vi "Send Delayed Set DER Control.vi"(5 "Message Type":refnum<class "Set DER Control Msg.lvclass">, 7 "Message Priority (Normal)":T3=enum."Normal", 8 "error in (no error)":errorcluster, 9 "Milliseconds To Wait":i32=1000, 10 "DER_Control":T1, 11 "Message Enqueuer":refnum<class "Message Enqueuer.lvclass">) -> (0 "error out":errorcluster, 3 "Message Enqueuer out":refnum<class "Message Enqueuer.lvclass">)   [LabVIEW 2018, in "Device Communication and Control Abstract Actor.lvlib" / "Set DER Control Msg.lvclass"]
doc: "This VI sends the message to an actor."
uses:
  Set DER Control Msg.lvclass
  <vilib>/ActorFramework/Message Enqueuer/Message Enqueuer.lvclass
  <vilib>/ActorFramework/Message Enqueuer/Message Priority.ctl
  C:/Program Files (x86)/National Instruments/LabVIEW 2018/vi.lib/ActorFramework/Message/Message.lvclass
  <vilib>/ORNL/CSEISMIC DDS/CSEISMIC DDS Base/Data Types/DER_Control.ctl
  <vilib>/ORNL/CSEISMIC DDS/CSEISMIC DDS Base/Data Types/Controls/DeviceID.ctl
  Set DER Control Msg.lvclass/Set DER Control Msg.ctl
  <vilib>/ORNL/CSEISMIC DDS/CSEISMIC DDS Base/CSEISMIC DDS.lvclass
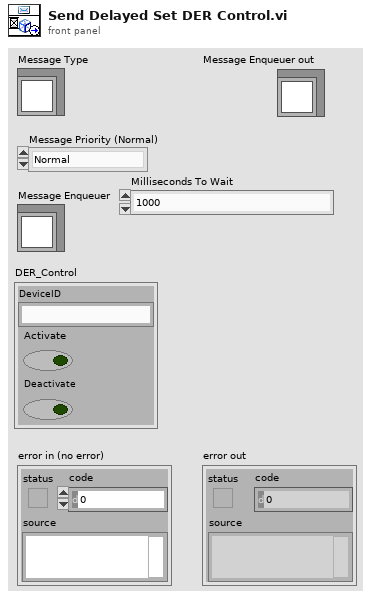
[diagram p1: front panel]
types:
  T1 = typedef "CSEISMIC DDS.lvlib/CSEISMIC DDS.lvclass/DER_Control.ctl" = cluster{"DeviceID":T2, "Activate":bool, "Deactivate":bool}
  T2 = typedef "CSEISMIC DDS.lvlib/CSEISMIC DDS.lvclass/DeviceID.ctl" = string
  T3 = typedef "Actor Framework.lvlib/Message Enqueuer.lvclass/Message Priority.ctl" = enum16{"Low", "Normal", "High"}
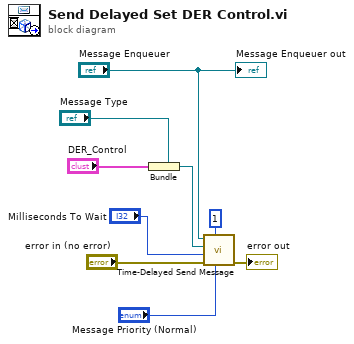
[diagram p0: block diagram]
diagram:
  n1 = Bundle(cluster="Message Type", "DER_Control") -> (w6:refnum<class "Set DER Control Msg.lvclass">)
  n2 = call <vilib>:"Time-Delayed Send Message.vi"("Message Priority (Normal)"="Message Priority (Normal)", "# Copies (0 = infinite repeat)"=u32 1, "error in (no error)"="error in (no error)", "Milliseconds To Wait"="Milliseconds To Wait", "Message"=w6, "Message Enqueuer"="Message Enqueuer") -> ("error out"=→"error out":errorcluster)  [unwired: 4 in, 1 out]
  "Message Enqueuer out" <- "Message Enqueuer"
